vi "Wait Notification.vi"(8 "error in (no error)":errorcluster, 9 "Timeout":i32, 11 "RT FIFO I64 Notifier in":refnum<class "RT FIFO I64 Notifier.lvclass">) -> (0 "error out":errorcluster, 1 "Timeout?":bool, 2 "Notification":variant, 3 "RT FIFO I64 Notifier out":refnum<class "RT FIFO I64 Notifier.lvclass">)   [LabVIEW 2022 SP3, in "RT FIFO I64 Notifier.lvclass"]
uses:
  RT FIFO I64 Notifier.lvclass
  RT FIFO I64 Notifier.lvclass/RT FIFO I64 Notifier.ctl
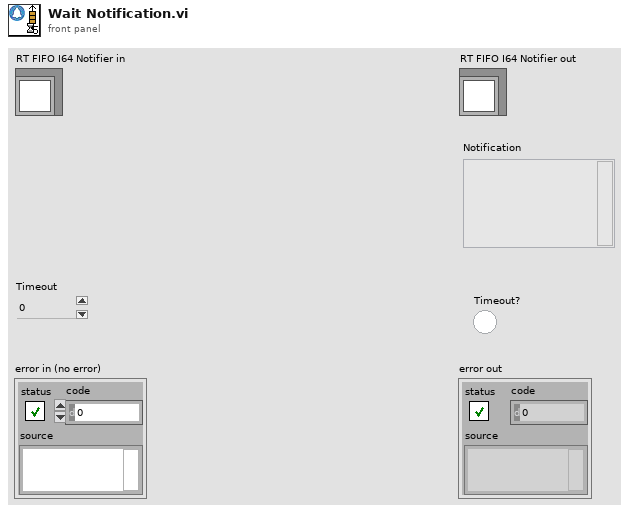
[diagram p1: front panel]
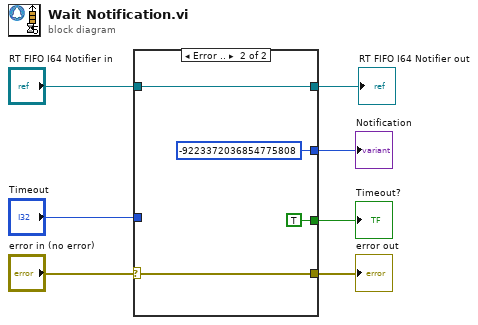
[diagram p0: block diagram]
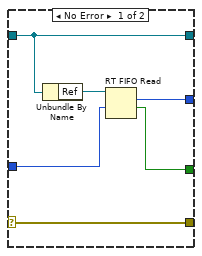
[diagram p2: hidden frame]
diagram:
  n1 = case shown="Error .." "error in (no error)" {
    selector: "error in (no error)" -> [w11 w17]
    tunnel: [w11 w17] -> w6
    tunnel: "RT FIFO I64 Notifier in" -> [w13 w16]
    tunnel: [w13 w16] -> w4
    tunnel: "Timeout" -> [w10 _]
    tunnel: [w9 i64 -9223372036854775808] -> w2
    tunnel: [w8 TRUE ("empty?")] -> w1
    frame No Error {
      n2 = Unbundle By Name(w13) -> ("Ref"=w12:refnum<k33>)
      n3 = RT FIFO Read(0:w12, 2:w10) -> (9:w9:i64, 10:w8:bool)  [unwired: 2 in, 3 out]
    }
    frame Error {
    }
  }
  "error out" <- w6
  "RT FIFO I64 Notifier out" <- w4
  "Notification" <- w2
  "Timeout?" <- w1
